vi "Redirector Test Select.vi"(11 "Error In":errorcluster) -> (4 "File Name":string, 6 "Subject Out":string, 8 "Delay":u32 max=1000 step=50, 10 "Interruptions":i32, 15 "Error Out":errorcluster)   [LabVIEW 2020, in "CollectionSupport.lvlib"]
uses:
  CollectionSupport.lvlib
panel:
  in  "Test Type":u16(ring) items=["Practice Run", "Normal", "Quiet"]
  in  "OK Button":bool
  in  "Subject":string
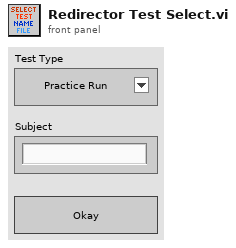
[diagram p1: front panel]
types:
  T1 = typedef "eventvkey.ctl" = enum16{"ASCII", "Enter", "Return", "Shift", "Ctrl", "Alt", "Cmd", "Opt", "Caps", "NumLock", "Clear", "Break", "Up", "Down", "Left", "Right", "Insert", "Delete", "Home", "End", "PageUp", "PageDown", "Escape", "Help", "Pause", "ScrollLock", "F1", "F2", "F3", "F4", "F5", "F6", "F7", "F8", "F9", "F10", "F11", "F12", "F13", "F14", "F15", "F16", "F17", "F18", "F19", "F20", "F21", "F22", "F23", "F24", "Play", "VolumeUp", "VolumeDown", "Mute", "Two Byte Char"}
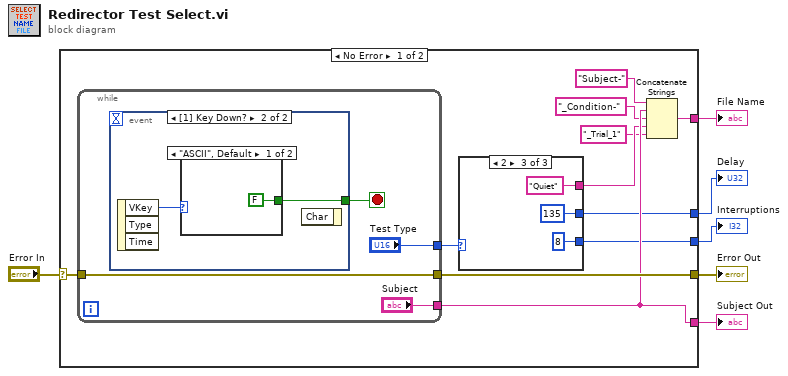
[diagram p0: block diagram]
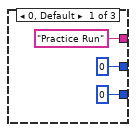
[diagram p2: hidden frame]
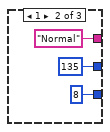
[diagram p3: hidden frame]
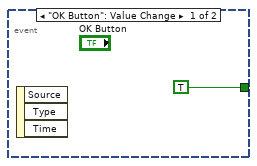
[diagram p4: hidden frame]
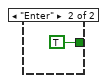
[diagram p5: hidden frame]
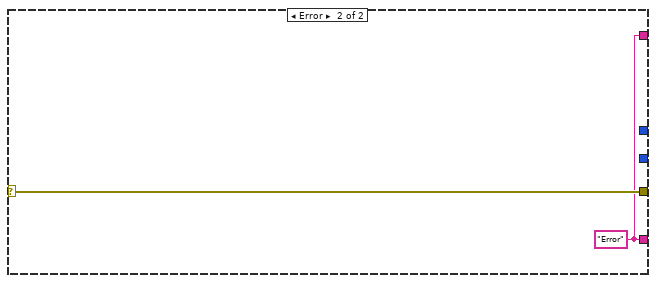
[diagram p6: hidden frame]
diagram:
  n1 = case shown="No Error" "Error In" {
    selector: "Error In" -> [w16 w37]
    tunnel: [w17 w37] -> w5
    tunnel: [w14 w36] -> w4
    tunnel: [w12 w36] -> w3
    tunnel: [w8 _] -> w2
    tunnel: [w7 _] -> w1
    frame No Error {
      n2 = while {
        tunnel: [w30] -> w17
        tunnel: w16 -> [w30]
        tunnel: ["Test Type"] -> w15
        tunnel: ["Subject"] -> w12
        stop <- w27 stop-if-true
        n3 = event shown="[1] Key Down?" {
          selector: _ -> [_ _]
          dyn-events: _ -> [_ _]
          timeout: _ -> [_ _]
          tunnel: [TRUE w32] -> w27
          event "OK Button": Value Change {
            n4 = event-data() -> ()  [unwired: 1 in, 3 out]
          }
          event Key Down? {
            n5 = event-data() -> ("VKey"=w33:T1)  [unwired: 1 in, 2 out]
            n6 = case shown="\"ASCII\", Default" w33 {
              tunnel: [FALSE TRUE] -> w32
              frame "ASCII", Default {
              }
              frame "Enter" {
              }
            }
            n7 = event-data() -> ()  [unwired: 2 in, 1 out]
          }
        }
      }
      n8 = case shown="2" w15 {
        tunnel: ["Practice Run" ("string") "Normal" ("string") "Quiet" ("string")] -> w10
        tunnel: [0 ("Interruptions") 8 ("Interruptions") 8 ("Interruptions")] -> w8
        tunnel: [u32 0 ("Delay") u32 135 ("Delay") u32 135 ("Delay")] -> w7
        frame 0, Default {
        }
        frame 1 {
        }
        frame 2 {
        }
      }
      n9 = Concatenate Strings("Subject-" ("default name"), w12, "_Condition-" ("string"), w10, "_Trial_1" ("string")) -> (w14:string)
    }
    frame Error {
      w36 = "Error"
    }
  }
  "Error Out" <- w5
  "File Name" <- w4
  "Subject Out" <- w3
  "Interruptions" <- w2
  "Delay" <- w1
